vi "RP Write Command.vi"   [LabVIEW 2015]
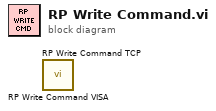
[diagram p0: block diagram]
diagram:
  n1 = call "RP Write Command VISA.vi"() -> ()  [unwired: 9 in, 3 out]
  n2 = call "RP Write Command TCP.vi"() -> ()  [unwired: 9 in, 3 out]
